vi "Line Plot.vi"() -> ()   [LabVIEW 2013]
uses:
  <vilib>/Heliosphere Research LLC/Advanced Plotting Toolkit/properties/Line.ctl
  <vilib>/Heliosphere Research LLC/Advanced Plotting Toolkit/properties/Line_Style.ctl
  <vilib>/Heliosphere Research LLC/Advanced Plotting Toolkit/typedefs/PlotColor.ctl
  <vilib>/Heliosphere Research LLC/Advanced Plotting Toolkit/properties/Marker.ctl
  <vilib>/Heliosphere Research LLC/Advanced Plotting Toolkit/properties/Marker_Style.ctl
  <vilib>/Heliosphere Research LLC/Advanced Plotting Toolkit/api_plotting/LineProperties.ctl
  <vilib>/Heliosphere Research LLC/Advanced Plotting Toolkit/properties/Display.ctl
  <vilib>/Heliosphere Research LLC/Advanced Plotting Toolkit/Advanced Plotting Toolkit.lvlib
panel:
  in  "Marker":T1={"Style"=enum."Square", "Color"=2147483647, "Size"=nan} {"Color" items=["Automatic"=2147483647, "Black"=0, "White"=16777215, "Red"=16711680, "Green"=2263842, "Blue"=255, "Cyan"=65535, "Magenta"=16711935, "Yellow"=16776960]}
  in  "Line":T4={"Style"=enum."Dashed", "Color"=2147483647, "Width"=nan} {"Color" items=["Automatic"=2147483647, "Black"=0, "White"=16777215, "Red"=16711680, "Green"=2263842, "Blue"=255, "Cyan"=65535, "Magenta"=16711935, "Yellow"=16776960]}
  out "Line Plot":picture
  # "Line Plots"
  # "Line plots are one of the simplest but most versatile elements\nin the Toolkit.  By default, a plain line is displayed, whose\ncolor is taken from the automatic color cycle.  \n\nYou can change the appearance of the line using the property\ncluster.  Try different settings below.  In this example, we've\nset the line style to Dashed and the marker style to Square.\nTry setting them back to Automatic to see what a default\nline looks like."
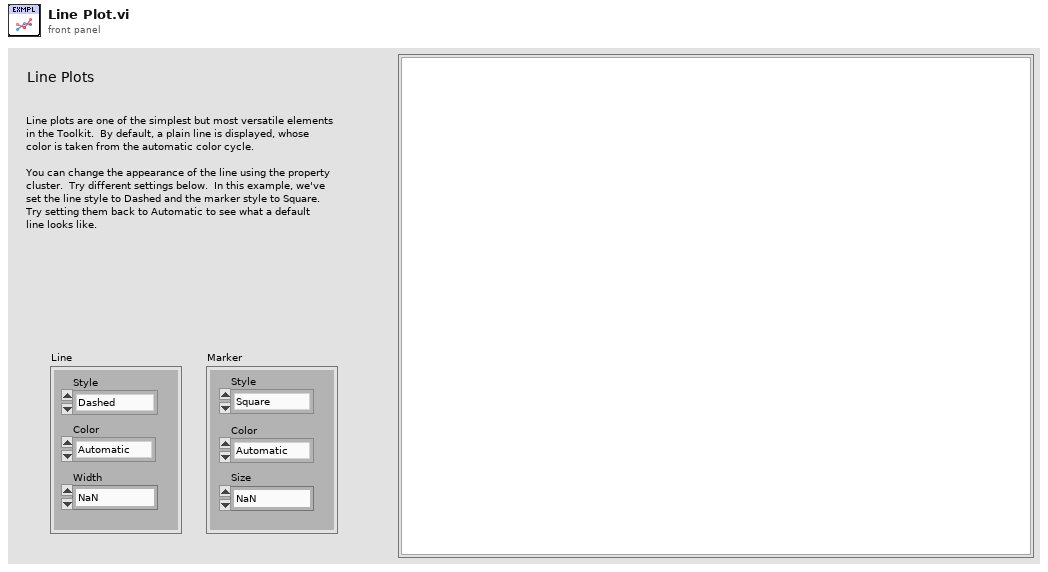
[diagram p1: front panel]
types:
  T1 = typedef "Advanced Plotting Toolkit.lvlib/Marker.ctl" = cluster{"Style":T2, "Color":T3, "Size":dbl}
  T2 = typedef "Advanced Plotting Toolkit.lvlib/Marker_Style.ctl" = enum16{"Automatic", "Circle", "Square", "Triangle", "Diamond", "Star", "Invisible"}
  T3 = typedef "Advanced Plotting Toolkit.lvlib/PlotColor.ctl" = u32
  T4 = typedef "Advanced Plotting Toolkit.lvlib/Line.ctl" = cluster{"Style":T5, "Color":T3, "Width":sgl}
  T5 = typedef "Advanced Plotting Toolkit.lvlib/Line_Style.ctl" = enum16{"Automatic", "Solid", "Dashed", "Dotted", "Dash-dot", "Invisible"}
  T6 = typedef "Advanced Plotting Toolkit.lvlib/LineProperties.ctl" = cluster{"Line":T4, "Marker":T1, "Display":T7}
  T7 = typedef "Advanced Plotting Toolkit.lvlib/Display.ctl" = cluster{"Alpha":dbl, "Z Order":dbl}
  T8 = typedef "Advanced Plotting Toolkit.lvlib/PlotID.ctl" = i32
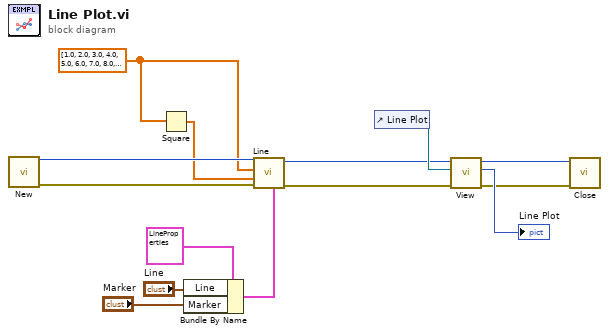
[diagram p0: block diagram]
diagram:
  w5 = dbl[] [1.0, 2.0, 3.0, 4.0, 5.0, 6.0, 7.0, 8.0, 9.0, 10.0] ("Y Data")
  n1 = call <vilib>:"New.vi"() -> ("error out"=w3:errorcluster, "Plot ID"=w11:T8)  [unwired: 10 in]
  n2 = Square(x=w5) -> (x^2=w4:dbl[])
  n3 = Bundle By Name(cluster=T6 {"Line"={"Style"=enum."Automatic", "Color"=2147483647, "Width"=nan}, "Marker"={"Style"=enum."Automatic", "Color"=2147483647, "Size"=nan}, "Display"={"Alpha"=nan, "Z Order"=nan}} ("Line Plot Properties"), "Line"="Line", "Marker"="Marker") -> (w8:T6)
  n4 = call <vilib>:"Line.vi"("Properties"=w8, "error in (no error)"=w3, "Y Data"=w4, "X Data"=w5, "Plot ID"=w11) -> ("error out"=w2:errorcluster, "Plot ID out"=w10:T8)  [unwired: 5 in]
  n5 = control-ref of="Line Plot"() -> (w14:refnum<vi>)
  n6 = call <vilib>:"View.vi"("error in (no error)"=w2, "Ref for Sizing"=w14, "Plot ID"=w10) -> ("error out"=w1:errorcluster, "Picture"=→"Line Plot":picture, "Plot ID Out"=w12:T8)  [unwired: 6 in]
  n7 = call <vilib>:"Close.vi"("error in (no error)"=w1, "Plot ID"=w12) -> ()  [unwired: 9 in, 1 out]
